vi "ElementAtGoalieArea.vi"(7 "Elemento pos.":dbl[](array[numeric]), 8 "error in (no error)":errorcluster, 10 "Game":refnum<class "Game.lvclass">, 11 "Utilities in":refnum<class "Utilities.lvclass">) -> (0 "error out":errorcluster, 2 "Elemento at goalkeeper area ?":bool, 3 "Utilities out":refnum<class "Utilities.lvclass">)   [LabVIEW 2018, in "Utilities.lvclass"]
uses:
  Utilities.lvclass
  Game_class/Game.lvclass
  Game_class/Game.lvclass/Game.ctl
  Parameters_class/Parameters.lvclass/Parameters.ctl
  Parameters_class/Read Area.vi
  Game_class/Read FieldRef.vi
  Game_class/Read Parameters.lvclass.vi
  Field_class/Field.lvclass
  Parameters_class/Parameters.lvclass
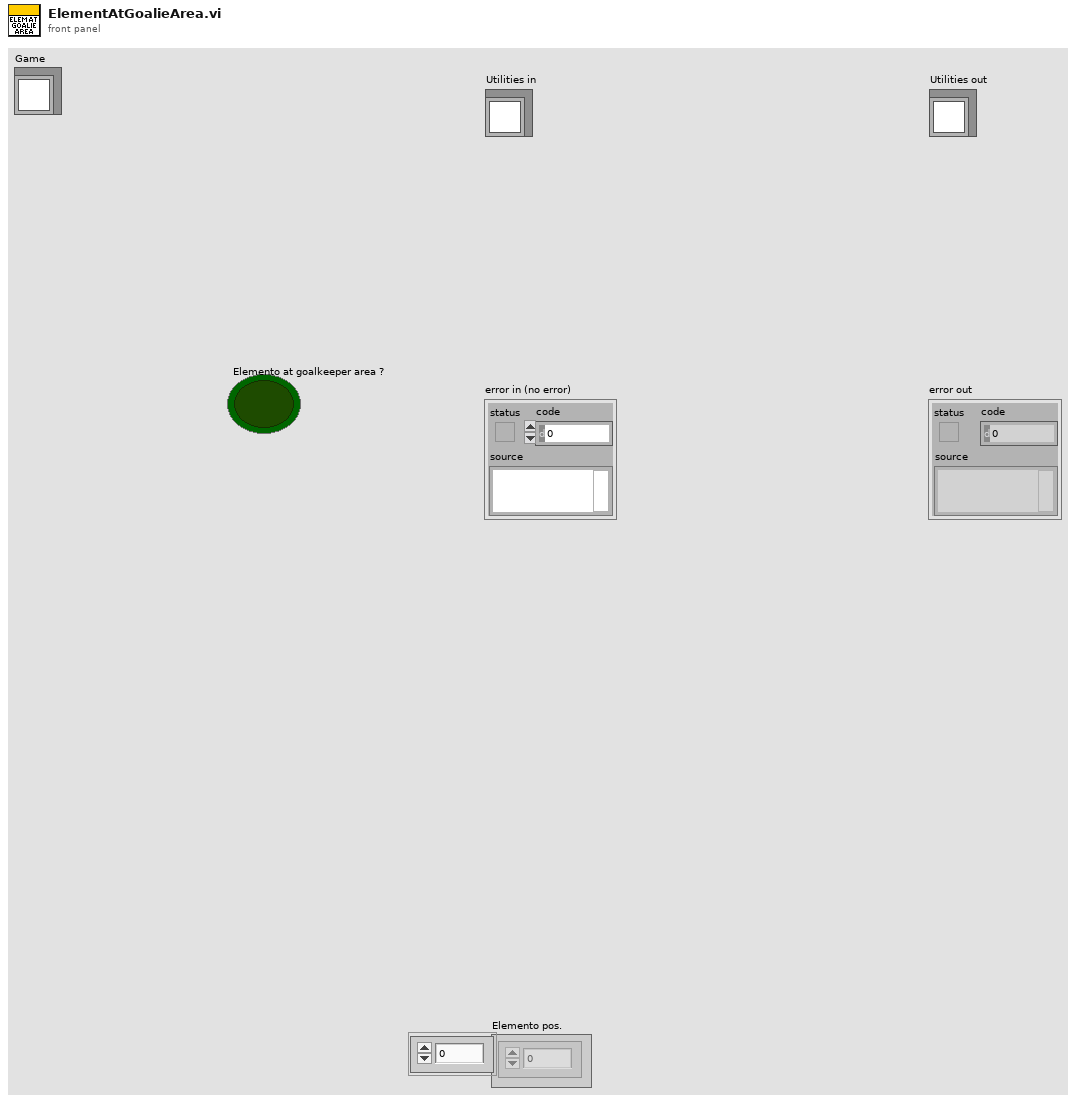
[diagram p1: front panel]
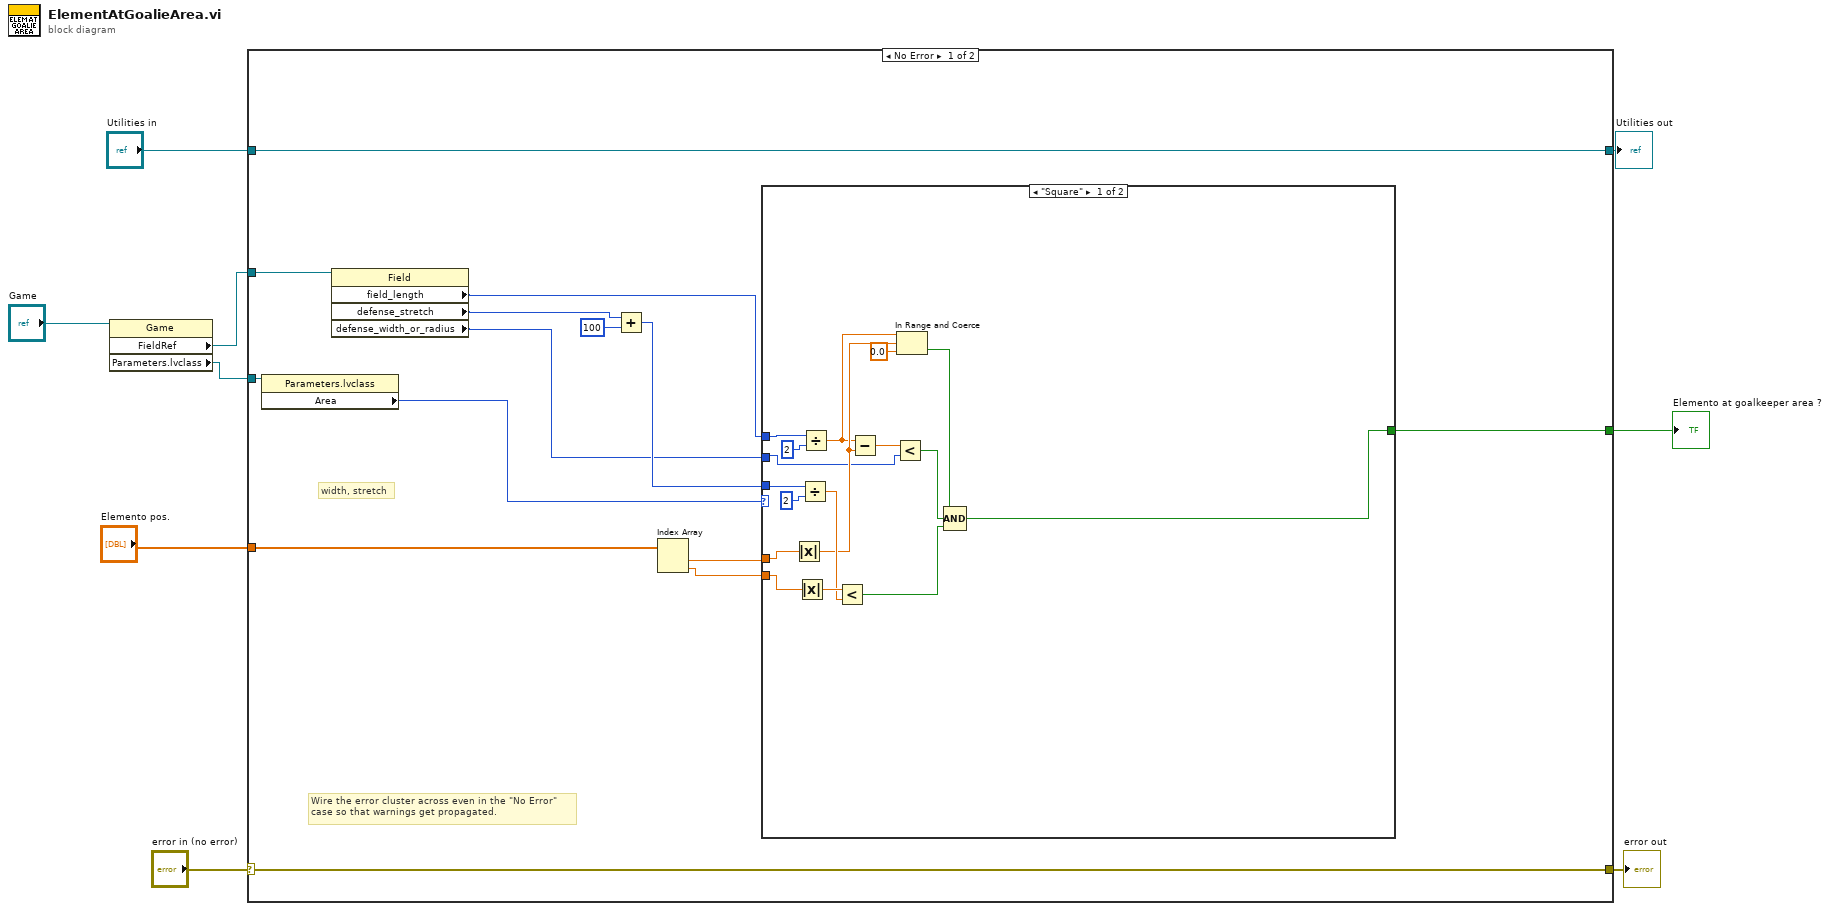
[diagram p0: block diagram]
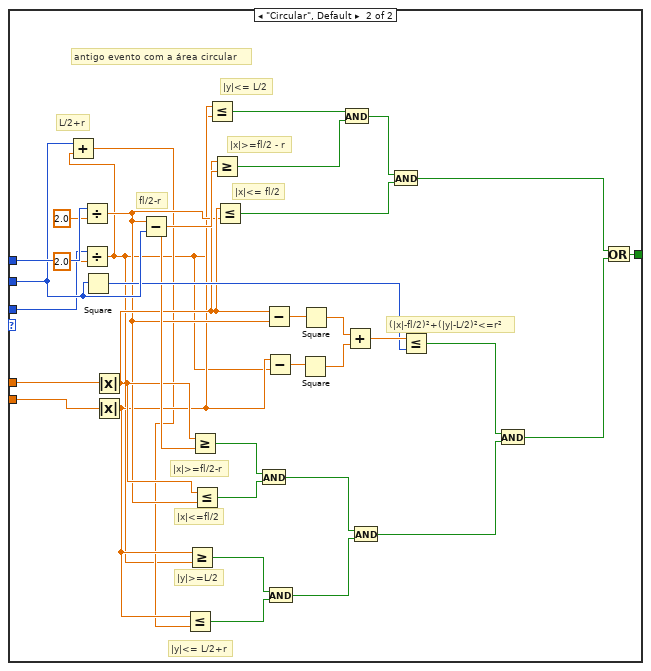
[diagram p2: hidden frame]
diagram:
  n1 = property class="Game"(reference="Game") -> ("FieldRef"=w3:refnum<class "Field.lvclass">, "Parameters.lvclass"=w2:refnum<class "Parameters.lvclass">)  [unwired: 1 in, 2 out]
  n2 = case shown="No Error" "error in (no error)" {
    selector: "error in (no error)" -> [w22 w76]
    tunnel: [w22 w76] -> w8
    tunnel: [w23 w75] -> w6
    tunnel: "Utilities in" -> [w23 w75]
    tunnel: w3 -> [w14 _]
    tunnel: "Elemento pos." -> [w13 _]
    tunnel: [w12 _] -> w4
    tunnel: w2 -> [w11 _]
    frame No Error {
      # "width, stretch"
      # "Wire the error cluster across even in the \"No Error\"\ncase so that warnings get propagated."
      n3 = property class="Parameters.lvclass"(reference=w11) -> ("Area"=w10:enum16{"Circular", "Square"})  [unwired: 1 in, 2 out]
      n4 = property class="Field"(reference=w14) -> ("field_length"=w17:i32, "defense_stretch"=w16:i32, "defense_width_or_radius"=w15:i32)  [unwired: 1 in, 2 out]
      n5 = Add(x=w16, y=u32 100) -> (x+y=w20:u32)
      n6 = Index Array(array=w13) -> (element #1=w18:dbl, element #2=w19:dbl)  [unwired: 2 in]
      n7 = case shown="\"Square\"" w10 {
        tunnel: w19 -> [w28 w74]
        tunnel: w18 -> [w29 w73]
        tunnel: w17 -> [w26 w72]
        tunnel: [w24 w71] -> w12
        tunnel: w15 -> [w25 w70]
        tunnel: w20 -> [w27 w69]
        frame "Square" {
          n8 = Absolute Value(x=w29) -> (abs(x)=w33:dbl)
          n9 = Absolute Value(x=w28) -> (abs(x)=w39:dbl)
          n10 = Divide(x=w27, y=u32 2) -> (x/y=w36:dbl)
          n11 = Divide(x=w26, y=u32 2) -> (x/y=w31:dbl)
          n12 = Less?(x=w39, y=w36) -> (x < y?=w34:bool)
          n13 = Subtract(x=w31, y=w33) -> (x-y=w38:dbl)
          n14 = Less?(x=w38, y=w25) -> (x < y?=w35:bool)
          n15 = In Range and Coerce(upper limit=w31, x=w33, lower limit=0.0) -> (In Range?=w30:bool)  [unwired: 1 out]
          n16 = Compound Arithmetic op=AND(w30, w35, w34) -> (w24:bool)
        }
        frame "Circular", Default {
          # "antigo evento com a área circular"
          # "|y|<= L/2+r"
          # "L/2+r"
          # "|y|>=L/2"
          # "|x|<=fl/2"
          # "|x|>=fl/2-r"
          # "fl/2-r"
          # "(|x|-fl/2)²+(|y|-L/2)²<=r²"
          # "|x|<= fl/2"
          # "|x|>=fl/2 - r"
          # "|y|<= L/2"
          n17 = Divide(x=w72, y=2.0) -> (x/y=w52:dbl)
          n18 = Divide(x=w69, y=2.0) -> (x/y=w41:dbl)
          n19 = Add(x=w70, y=w41) -> (x+y=w50:dbl)
          n20 = Square(x=w70) -> (x^2=w57:i32)
          n21 = Absolute Value(x=w73) -> (abs(x)=w55:dbl)
          n22 = Absolute Value(x=w74) -> (abs(x)=w51:dbl)
          n23 = Subtract(x=w52, y=w70) -> (x-y=w56:dbl)
          n24 = Less Or Equal?(x=w51, y=w50) -> (x <= y?=w48:bool)
          n25 = Greater Or Equal?(x=w51, y=w41) -> (x >= y?=w49:bool)
          n26 = Greater Or Equal?(x=w55, y=w56) -> (x >= y?=w54:bool)
          n27 = Less Or Equal?(x=w55, y=w52) -> (x <= y?=w53:bool)
          n28 = Less Or Equal?(x=w51, y=w41) -> (x <= y?=w66:bool)
          n29 = Greater Or Equal?(x=w55, y=w56) -> (x >= y?=w65:bool)
          n30 = Less Or Equal?(x=w55, y=w52) -> (x <= y?=w63:bool)
          n31 = And(x=w54, y=w53) -> (x .and. y?=w47:bool)
          n32 = Subtract(x=w55, y=w52) -> (x-y=w62:dbl)
          n33 = Subtract(x=w51, y=w41) -> (x-y=w61:dbl)
          n34 = And(x=w49, y=w48) -> (x .and. y?=w46:bool)
          n35 = Square(x=w61) -> (x^2=w59:dbl)
          n36 = Square(x=w62) -> (x^2=w60:dbl)
          n37 = And(x=w66, y=w65) -> (x .and. y?=w64:bool)
          n38 = Add(x=w60, y=w59) -> (x+y=w58:dbl)
          n39 = And(x=w47, y=w46) -> (x .and. y?=w44:bool)
          n40 = And(x=w64, y=w63) -> (x .and. y?=w43:bool)
          n41 = Less Or Equal?(x=w58, y=w57) -> (x <= y?=w45:bool)
          n42 = And(x=w45, y=w44) -> (x .and. y?=w42:bool)
          n43 = Or(x=w43, y=w42) -> (x .or. y?=w71:bool)
        }
      }
    }
    frame Error {
    }
  }
  "error out" <- w8
  "Utilities out" <- w6
  "Elemento at goalkeeper area ?" <- w4
